vi "PAM Create Save Directory.vi"() -> (0 "Error Out":errorcluster, 3 "Path":path)   [LabVIEW 2020]
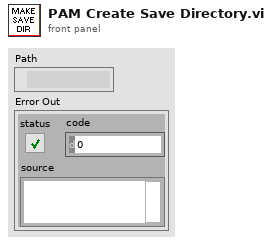
[diagram p1: front panel]
types:
  T1 = cluster{"Time Window":dbl, "Base Folder Path":path, "Collect Training Frames?":bool}
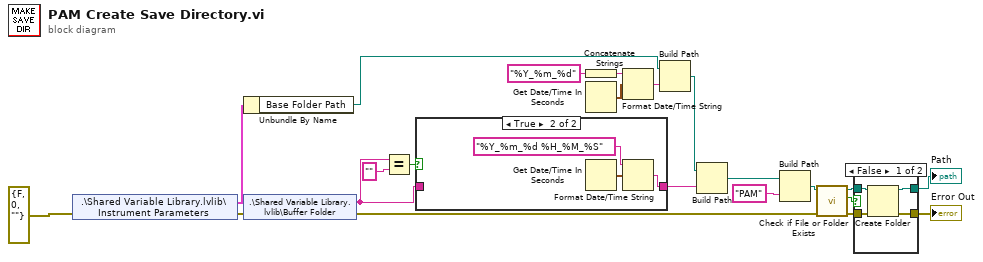
[diagram p0: block diagram]
diagram:
  n1 = shared-variable ".\\Shared Variable Library.lvlib\\Instrument Parameters"(error in=errorcluster {"status"=FALSE, "code"=0, "source"=""} ("Error In")) -> (w19:T1, error out=w13:errorcluster)
  n2 = Unbundle By Name(w19) -> ("Base Folder Path"=w1:path)
  n3 = shared-variable ".\\Shared Variable Library.lvlib\\Buffer Folder"(error in=w13) -> (w10:string, error out=w5:errorcluster)
  n4 = Equal?(x=w10, y="" ("Buffer Folder")) -> (x = y?=w11:bool)
  n5 = case shown="True" w11 {
    tunnel: [w23 w25] -> w9
    tunnel: w10 -> [w23 _]
    frame False {
    }
    frame True {
      n6 = Get Date/Time In Seconds() -> (seconds since 1Jan1904=w26:timestamp)
      n7 = Format Date/Time String(time format string (%c)="%Y_%m_%d %H_%M_%S", seconds (now)=w26) -> (date/time string=w25:string)  [unwired: 1 in]
    }
  }
  n8 = Concatenate Strings("%Y_%m_%d" ("time format string (%c)")) -> (w22:string)
  n9 = Get Date/Time In Seconds() -> (seconds since 1Jan1904=w20:timestamp)
  n10 = Format Date/Time String(time format string (%c)=w22, seconds (now)=w20) -> (date/time string=w17:string)  [unwired: 1 in]
  n11 = Build Path(base path=w1, name or relative path=w17) -> (appended path=w15:path)
  n12 = Build Path(base path=w15, name or relative path=w9) -> (appended path=w14:path)
  n13 = Build Path(base path=w14, name or relative path="PAM") -> (appended path=w4:path)
  n14 = call <vilib>:"Check if File or Folder Exists.vi"("error in (no error)"=w5, "path"=w4) -> ("error out"=w8:errorcluster, "file or folder exists?"=w6:bool, "dup path"=w7:path)  [unwired: 7 in]
  n15 = case shown="False" w6 {
    tunnel: [w30 w32] -> w3
    tunnel: w7 -> [w29 w32]
    tunnel: w8 -> [w28 w31]
    tunnel: [w27 w31] -> w2
    frame False {
      n16 = Create Folder(path (use dialog)=w29, error in=w28) -> (created path=w30:path, error out=w27:errorcluster)  [unwired: 1 in, 1 out]
    }
    frame True {
    }
  }
  "Path" <- w3
  "Error Out" <- w2
